vi "Stop Undo.vi"(8 "error in (no error)":errorcluster, 11 "CSM-Helper in":refnum<class "CSM-Helper.lvclass">) -> (0 "error out":errorcluster, 3 "CSM-Helper out":refnum<class "CSM-Helper.lvclass">)   [LabVIEW 2017, in "CSM-Helper.lvclass"]
doc: "### Stop Undo.vi\n\n-- <b>Controls</b> --\n- <b>CSM-Helper in</b>: CSMHelper input\n\n-- <b>Indicators</b> --\n- <b>CSM-Helper out</b>: CSMHelper output"
uses:
  CSM-Helper.lvclass
  CSM-Helper.lvclass/CSM-Helper.ctl
  Properties/Read VI Ref.vi
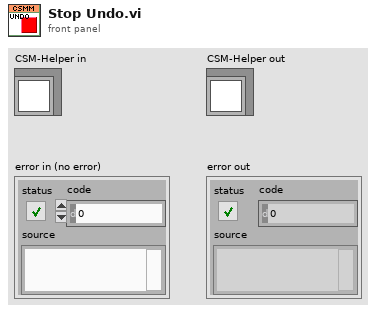
[diagram p1: front panel]
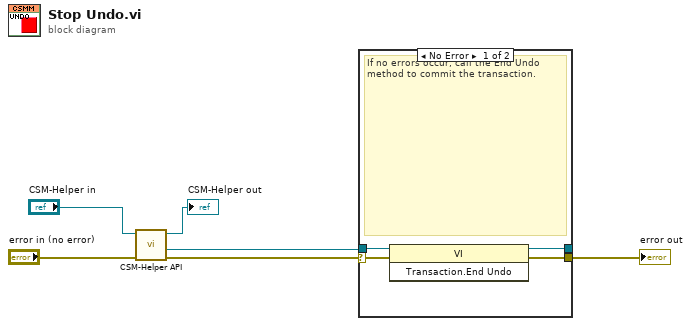
[diagram p0: block diagram]
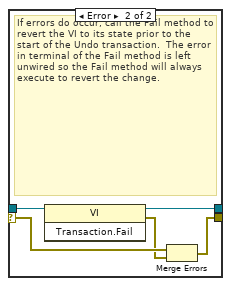
[diagram p2: hidden frame]
diagram:
  n1 = call-poly "CSM-Helper API.vi"("error in (no error)"="error in (no error)", "CSM-Helper in"="CSM-Helper in") -> ("error out"=w2:errorcluster, "VI"=w1:refnum<vi>, "CSM-Helper out"=→"CSM-Helper out":refnum<class "CSM-Helper.lvclass">)  [unwired: 7 in]
  n2 = case shown="No Error" w2 {
    selector: w2 -> [w9 w13]
    tunnel: w1 -> [w10 w15]
    tunnel: [w8 w14] -> _
    tunnel: [w7 w11] -> w3
    frame No Error {
      # "If no errors occur, call the End Undo method to commit the transaction."
      n3 = invoke class="VI" method="Transaction.End Undo"(reference=w10, error in=w9) -> (reference out=w8:refnum<vi>, error out=w7:errorcluster)  [unwired: 1 in, 1 out]
    }
    frame Error {
      # "If errors do occur, call the Fail method to revert the VI to its state prior to the start of the Undo transaction.  The error in terminal of the Fail method is left unwired so the Fail method will always execute to revert the change."
      n4 = invoke class="VI" method="Transaction.Fail"(reference=w15) -> (reference out=w14:refnum<vi>, error out=w12:errorcluster)  [unwired: 2 in, 1 out]
      n5 = Merge Errors(w13, w12) -> (w11:errorcluster)
    }
  }
  "error out" <- w3
